vi "Get Picture.vi"(8 "error in (no error)":errorcluster, 11 "Novatech in":refnum<class "Novatech.lvclass">) -> (0 "error out":errorcluster, 2 "Device Pic":T1, 3 "Novatech out":refnum<class "Novatech.lvclass">)   [LabVIEW 2013, in "Novatech.lvclass"]
uses:
  Novatech.lvclass
  <vilib>/picture/picture.llb/imagedata.ctl
panel:
  in  "path to PNG file":path=path "C:/Users/Zack/Dropbox/LabView_SetListRewrite/TableTest/DeviceVIs/Novatech/novatech.png"
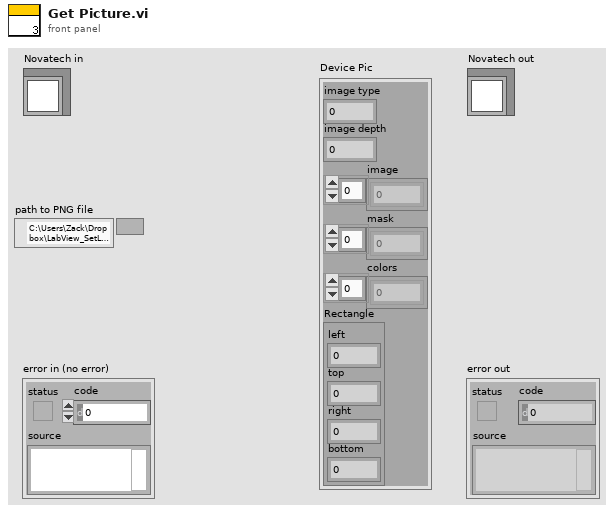
[diagram p1: front panel]
types:
  T1 = typedef "imagedata.ctl" = cluster{"image type":i32, "image depth":i32, "image":u8[], "mask":u8[], "colors":u32[], "Rectangle":cluster{"left":i16, "top":i16, "right":i16, "bottom":i16}}
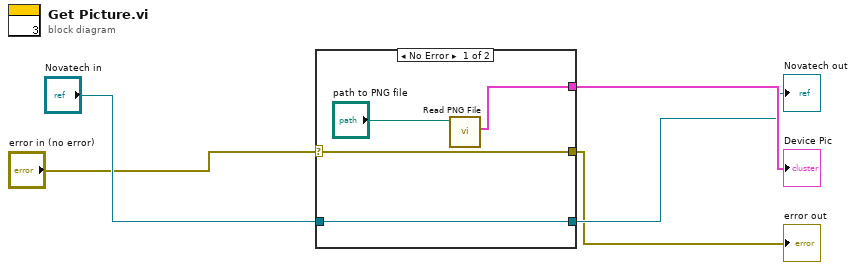
[diagram p0: block diagram]
diagram:
  n1 = case shown="No Error" "error in (no error)" {
    selector: "error in (no error)" -> [w8 w10]
    tunnel: [w8 w10] -> w1
    tunnel: [w7 w11] -> w2
    tunnel: "Novatech in" -> [w7 w11]
    tunnel: [w6 _] -> w3
    frame No Error {
      n2 = call <vilib>:"Read PNG File.vi"("path to PNG file"="path to PNG file") -> ("image data"=w6:T1)  [unwired: 8 in, 2 out]
    }
    frame Error {
    }
  }
  "error out" <- w1
  "Novatech out" <- w2
  "Device Pic" <- w3
